vi "Equalize.vi"(0 "Input Image":T1={"Image ID"=0, "Channel ID"=-1}, 1 "Output Image":T1={"Image ID"=0, "Channel ID"=-1}, 2 "Minimum":u8, 3 "Maximum":u8, 4 "Error":string) -> (5 "Input Image":T1={"Image ID"=0, "Channel ID"=-1}, 6 "Output Image":T1={"Image ID"=0, "Channel ID"=-1}, 7 "Error":string)   [LabVIEW 2011, in "labvvis.lvlib"]
doc: "Equalise distributes the grey-level interval (Minimum to Maximum) evenly over the full grey scale (0 to 255).\n\nThe result of any pixel which is less than or equal to Minimum is 0. For pixels larger than Maximum, the result is 255. For any other pixel, the result is adjusted using a linear equation."
uses:
  <userlib>/labvvis/labvvis.lvlib
  <userlib>/labvvis/VVIS Image.ctl
  labvvis.framework
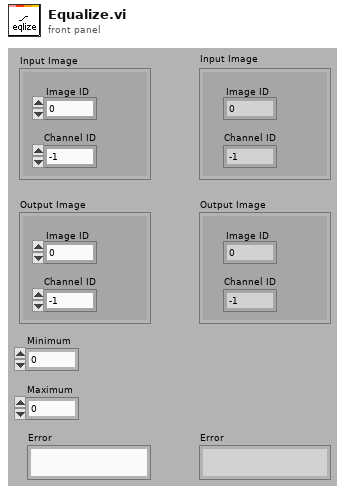
[diagram p1: front panel]
types:
  T1 = typedef "labvvis.lvlib/VVIS Image.ctl" = cluster{"Image ID":i16, "Channel ID":i16}
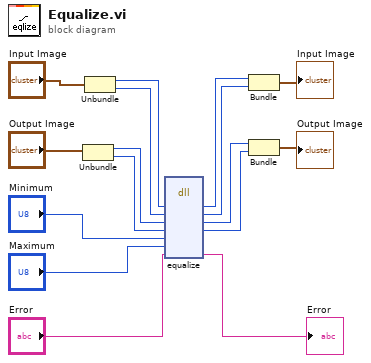
[diagram p0: block diagram]
diagram:
  n1 = Unbundle("Output Image") -> ("Image ID"=w12:i16, "Channel ID"=w11:i16)
  n2 = Unbundle("Input Image") -> ("Image ID"=w14:i16, "Channel ID"=w13:i16)
  n3 = dll-call lib="labvvis.framework" fn="equalize"("src1"=w14, "icid"=w13, "out"=w12, "ocid"=w11, "min"="Minimum", "max"="Maximum", "Error") -> ("src1"=w3:i16, "icid"=w4:i16, "out"=w5:i16, "ocid"=w6:i16, →"Error":string)  [unwired: 6 in, 2 out]
  n4 = Bundle("src1"=w3, "icid"=w4) -> (→"Input Image":cluster{"src1":i16, "icid":i16})  [unwired: 1 in]
  n5 = Bundle("out"=w5, "ocid"=w6) -> (→"Output Image":cluster{"out":i16, "ocid":i16})  [unwired: 1 in]
